vi "LoadSimData.vi"(11 "filename":string) -> (3 "data":sgl[][](array[numeric]))   [LabVIEW 2017, in "IrAcquisition.lvlib"]
uses:
  <vilib>/addons/InsightCM/Devices/Shared/Ir/IrAcquisition/IrAcquisition.lvlib
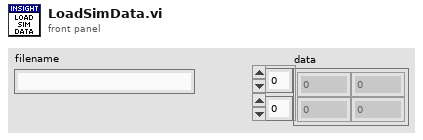
[diagram p1: front panel]
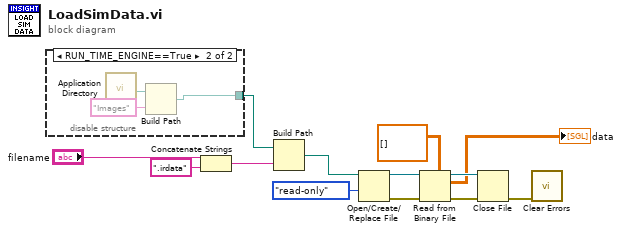
[diagram p0: block diagram]
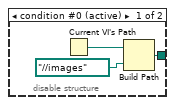
[diagram p2: hidden frame]
diagram:
  n1 = disable-structure shown="RUN_TIME_ENGINE==True" {
    disable-tunnel: [w14 w18] -> w11
    frame condition #0 (active) {
      n2 = Current VI's Path() -> (path=w16:path)
      n3 = Build Path(base path=w16, name or relative path=path "../../images" ("path")) -> (appended path=w14:path)
    }
    frame condition #1 {
      n4 = call <vilib>:"Application Directory.vi"() -> ("Application Directory"=w19:path)
      n5 = Build Path(base path=w19, name or relative path="Images") -> (appended path=w18:path)
    }
  }
  n6 = Concatenate Strings("filename", ".irdata" ("string")) -> (w10:string)
  n7 = Build Path(base path=w11, name or relative path=w10) -> (appended path=w9:path)
  n8 = Open/Create/Replace File(file path (use dialog)=w9, access (0:read/write)=enum16{"read/write", "read-only", "write-only"}."read-only") -> (refnum out=w7:refnum<file>, error out=w6:errorcluster)  [unwired: 4 in, 1 out]
  n9 = Read from Binary File(5:sgl[][] [] ("data"), 8:w6, 11:w7) -> (0:w5:errorcluster, 2:→"data":sgl[][], 3:w8:refnum<file>)  [unwired: 3 in, 1 out]
  n10 = Close File(refnum=w8, error in=w5) -> (error out=w1:errorcluster)  [unwired: 1 out]
  n11 = call <vilib>:"Clear Errors.vi"("error in (no error)"=w1) -> ()  [unwired: 5 in, 2 out]
